vi "Digital Open.vi"(8 "Error In":errorcluster, 10 "Pins":u8[](array[numeric]), 11 "LINX Resource":T1) -> (0 "Error Out":errorcluster, 3 "LINX Resource":T1)   [LabVIEW 2011, in "LVH-LINX.lvlib"]
uses:
  LVH-LINX.lvlib
  Private/Type Defs/LINX Ref.ctl
  Private/Type Defs/Platform.ctl
  Private/Type Defs/Interface.ctl
  Private/Type Defs/TCP Config.ctl
  Private/Type Defs/LINX Device Config.ctl
panel:
  # "Pass in DIO pins and directions\nFor LINX set directions\nFor myRIO open pins, no need to set directions"
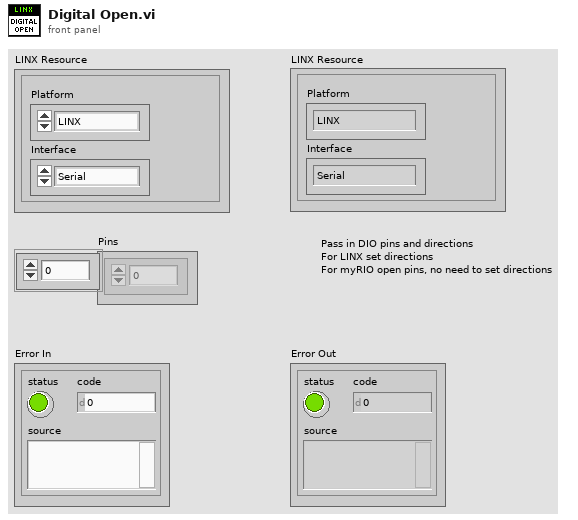
[diagram p1: front panel]
types:
  T1 = typedef "LVH-LINX.lvlib/LINX Ref.ctl" = cluster{"Platform":T2, "Interface":T3, "TCP Configuration":T4, "COM Port":refnum<visa-resource-name>, "LINX Device Config":T5}
  T2 = typedef "LVH-LINX.lvlib/Platform.ctl" = enum16{"LINX", "myRIO"}
  T3 = typedef "LVH-LINX.lvlib/Interface.ctl" = enum16{"Serial", "TCP"}
  T4 = typedef "LVH-LINX.lvlib/TCP Config.ctl" = cluster{"IP Address":string, "Port":dbl}
  T5 = typedef "LVH-LINX.lvlib/LINX Device Config.ctl" = cluster{"Interface":T3, "COM Port":refnum<visa-resource-name>, "Packet Number":u16, "TCP Configuration":T4}
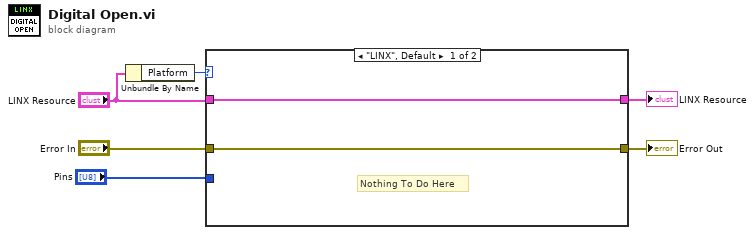
[diagram p0: block diagram]
diagram:
  n1 = Unbundle By Name("LINX Resource") -> ("Platform"=w6:T2)
  n2 = case shown="\"LINX\", Default" w6 {
    tunnel: "Error In" -> [w7 w9]
    tunnel: "LINX Resource" -> [w8 w10]
    tunnel: [w7 w9] -> w3
    tunnel: "Pins" -> [_ _]
    tunnel: [w8 w10] -> w2
    frame "LINX", Default {
      # "Nothing To Do Here"
    }
    frame "myRIO" {
      # "Add myRIO Stuff Here!!!"
    }
  }
  "Error Out" <- w3
  "LINX Resource" <- w2
